vi "digital_IO_test.vi"() -> ()   [LabVIEW 2017]
panel:
  out "Waveform Chart 2":dynamicdata(graph)
  out "Waveform Chart":dynamicdata(graph)
  in  "stop":bool
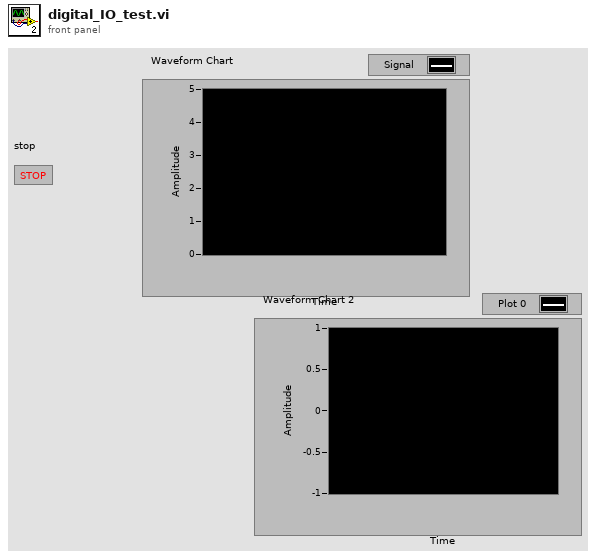
[diagram p1: front panel]
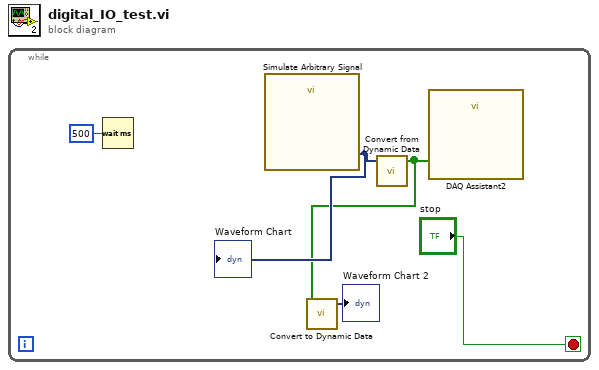
[diagram p0: block diagram]
diagram:
  n1 = while {
    stop <- "stop" stop-if-true
    n2 = Wait (ms)(milliseconds to wait=u32 500) -> ()  [unwired: 1 out]
    n3 = call "Simulate Arbitrary Signal"() -> ("Signal"=w3:dynamicdata)  [unwired: 9 in, 2 out]
    "Waveform Chart" <- w3
    n4 = call "Convert from Dynamic Data"("Dynamic Data Type"=w3) -> ("Array"=w2:bool[])  [unwired: 3 in]
    n5 = call "Convert to Dynamic Data"("Array"=w2) -> ("Dynamic Data Type"=→"Waveform Chart 2":dynamicdata)  [unwired: 3 in]
    n6 = call "DAQ Assistant2"("data"=w2) -> ()  [unwired: 17 in, 2 out]
  }
